vi "BTK current.vi"(9 "f factor":dbl[](array[numeric]), 10 "z factor":dbl[](array[numeric])) -> (2 "I current":dbl)   [LabVIEW 2021]
uses:
  <vilib>/Analysis/2dsp.llb/Integral Method.ctl
  <vilib>/Analysis/8numeric.llb/1D Numeric Integration.vi
  <vilib>/Analysis/NI_AALPro.lvlib
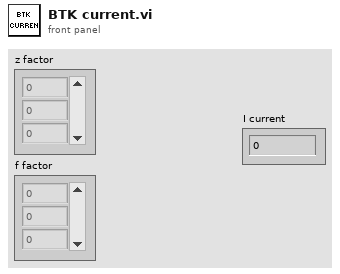
[diagram p1: front panel]
types:
  T1 = typedef "NI_AALPro.lvlib/Integral Method.ctl" = i32
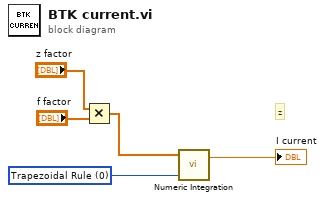
[diagram p0: block diagram]
diagram:
  w1 = T1 0 items=["Trapezoidal Rule", "Simpson's Rule", "Simpson's 3/8 Rule", "Bode Rule"] ("integration method")
  # "z"
  n1 = Multiply(x="z factor", y="f factor") -> (x*y=w3:dbl[])
  n2 = call-poly <vilib>:"Numeric Integration.vi"("integration method"=w1, "Input Array"=w3) -> ("result"=→"I current":dbl)  [unwired: 1 in, 1 out]
